vi "SW_Load_frames_from_XML_GL.vi"(2 "Input XML string":string) -> (0 "Output array of clusters with dataframes":T1(array[cluster]))   [LabVIEW 2016]
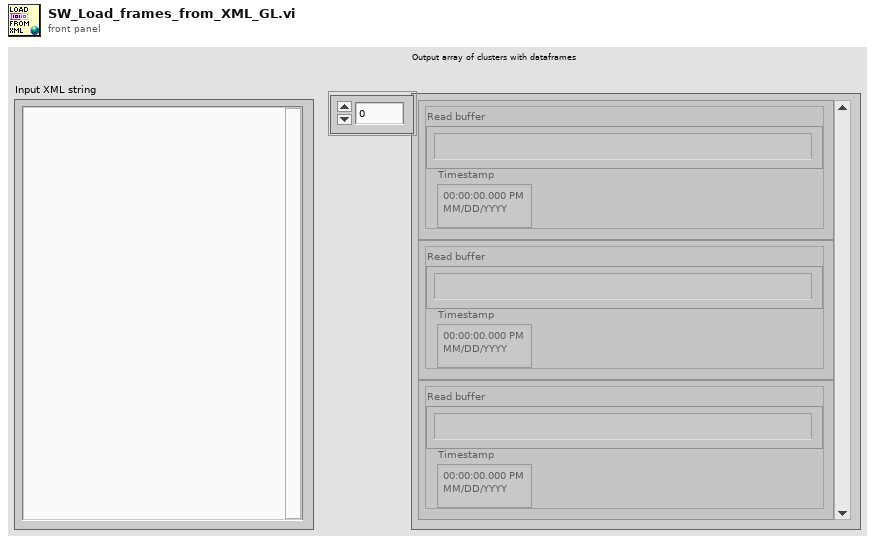
[diagram p1: front panel]
types:
  T1 = cluster{"Read buffer":string, "Timestamp":timestamp}[]
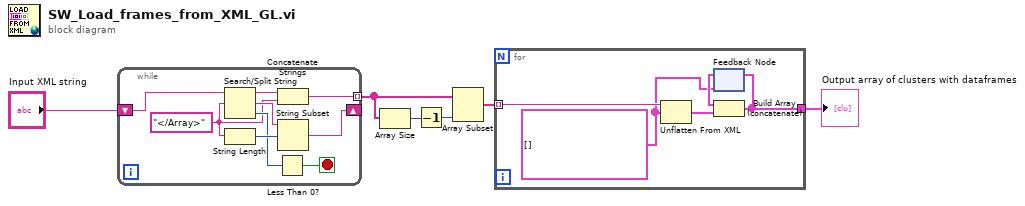
[diagram p0: block diagram]
diagram:
  n1 = while {
    shift-right: [w12] -> _
    shift-left: "Input XML string" -> [w15]
    tunnel: [w8] -> w2 mode=indexing
    stop <- w10 stop-if-true
    w7 = "</Array>" ("search string/char (-)")
    n2 = Search/Split String(string=w15, search string/char (-)=w7) -> (substring before match=w9:string, match + rest of string=w13:string, offset of match=w11:i32)  [unwired: 1 in]
    n3 = String Length(string=w7) -> (length=w14:i32)
    n4 = Less Than 0?(x=w11) -> (x < 0?=w10:bool)
    n5 = Concatenate Strings(w9, w7) -> (w8:string)
    n6 = String Subset(string=w13, offset (0)=w14) -> (substring=w12:string)  [unwired: 1 in]
  }
  n7 = Array Size(array=w2) -> (size(s)=w3:i32)
  n8 = Decrement(x=w3) -> (x-1=w4:i32)
  n9 = Array Subset(array=w2, length=w4) -> (w5:string[])  [unwired: 1 in]
  n10 = for {
    tunnel: w5 -> [w20] mode=indexing
    tunnel: [w16] -> w6
    w17 = T1 []
    n11 = Unflatten From XML(xml string=w20, type=w17) -> (value=w19:T1)  [unwired: 1 in, 1 out]
    n12 = feedback #1(w17) -> (w18:T1)
    n13 = Build Array (concatenate)(w18, w19) -> (w16:T1)
    n14 = feedback-in #1(w16) -> ()
  }
  "Output array of clusters with dataframes" <- w6
